vi "SaveData.vi"   [LabVIEW 2019]
types:
  T1 = enum16{"open", "replace", "create", "open or create", "replace or create", "replace or create with confirmation"}
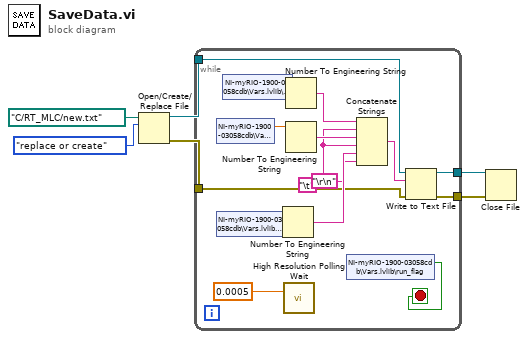
[diagram p0: block diagram]
diagram:
  n1 = Open/Create/Replace File(file path (use dialog)=path "C:/RT_MLC/new.txt", operation (0:open)=T1."replace or create") -> (refnum out=w4:refnum<file>, error out=w3:errorcluster)  [unwired: 4 in, 1 out]
  n2 = while {
    tunnel: w3 -> [w11]
    tunnel: w4 -> [w10]
    tunnel: [w9] -> w5
    tunnel: [w8] -> w6
    stop <- w7 stop-if-true
    w13 = "\t"
    n3 = shared-variable "NI-myRIO-1900-03058cdb\\Vars.lvlib\\dx"() -> (w16:dbl)  [unwired: 1 in, 1 out]
    n4 = shared-variable "NI-myRIO-1900-03058cdb\\Vars.lvlib\\u[A]"() -> (w14:dbl)  [unwired: 1 in, 1 out]
    n5 = shared-variable "NI-myRIO-1900-03058cdb\\Vars.lvlib\\x[m]"() -> (w18:dbl)  [unwired: 1 in, 1 out]
    n6 = Number To Engineering String(4:w14) -> (0:w15:string)  [unwired: 3 in]
    n7 = call <vilib>:"High Resolution Polling Wait.vi"("seconds to wait"=0.0005 ("Delay Time (s)")) -> ()  [unwired: 10 in, 1 out]
    n8 = Number To Engineering String(4:w18) -> (0:w19:string)  [unwired: 3 in]
    n9 = Number To Engineering String(4:w16) -> (0:w17:string)  [unwired: 3 in]
    n10 = shared-variable "NI-myRIO-1900-03058cdb\\Vars.lvlib\\run_flag"() -> (w7:bool)  [unwired: 1 in, 1 out]
    n11 = Concatenate Strings(w19, w13, w17, w13, w15, "\r\n") -> (w20:string)
    n12 = Write to Text File(file (use dialog)=w10, text=w20, error in=w11) -> (refnum out=w8:refnum<file>, error out=w9:errorcluster)  [unwired: 1 in, 1 out]
  }
  n13 = Close File(refnum=w6, error in=w5) -> ()  [unwired: 2 out]
